vi "Test Array Add.vi"() -> ()   [LabVIEW 2021]
uses:
  Source/Variable/Double Float/Double Float.lvclass
  Source/Variable/Double Float Array/Double Float Array 1D.lvclass
  C:/Users/Tim/Documents/LabVIEW/2021/Data Classes/Source/Element/Vector Parent/Vector Parent.lvclass
  Source/Element/Vector Parent/Vector Parent.lvclass/Vector Parent.ctl
  Source/Element/Vector Parent/Properties/Write Size.vi
  Source/Element/Vector Parent/Properties/Read Index.vi
panel:
  out "Index":i32
  out "Valid Index":bool
  in  "Numeric 2":dbl=1.0
  out "Numeric":dbl
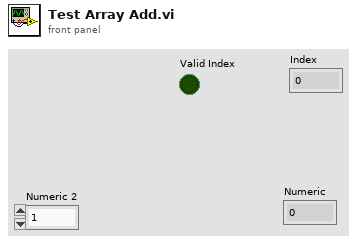
[diagram p1: front panel]
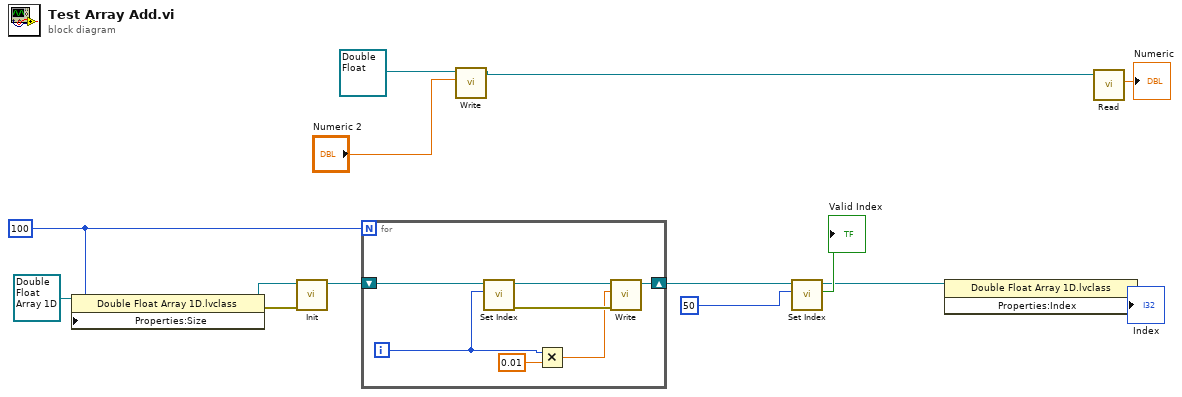
[diagram p0: block diagram]
diagram:
  w5 = 100
  n1 = property class="Double Float Array 1D.lvclass"(reference=refnum<class "Double Float Array 1D.lvclass"> refnum ("Variable.lvlib:Numeric Array.lvclass"), "Properties:Size"=w5) -> (reference out=w6:refnum<class "Double Float Array 1D.lvclass">, error out=w8:errorcluster)  [unwired: 1 in]
  n2 = call-dynamic "Init.vi"("error in (no error)"=w8, "Data in"=w6) -> ("Data out"=w11:refnum<class "Double Float Array 1D.lvclass">)  [unwired: 8 in, 1 out]
  n3 = for {
    N: w5 -> [_]
    shift-right: [w21] -> w10
    shift-left: w11 -> [w20]
    i -> [w17]
    n4 = call-dynamic "Set Index.vi"("Index"=w17, "Array in"=w20) -> ("error out"=w18:errorcluster, "Array out"=w19:refnum<class "Double Float Array 1D.lvclass">)  [unwired: 7 in, 1 out]
    n5 = Multiply(x=w17, y=0.01) -> (x*y=w15:dbl)
    n6 = call-dynamic "Write.vi"("error in (no error)"=w18, "Numeric"=w15, "Numeric Array in"=w19) -> ("Numeric Array out"=w21:refnum<class "Double Float Array 1D.lvclass">)  [unwired: 7 in, 1 out]
  }
  n7 = call-dynamic "Write.vi"("Numeric"="Numeric 2", "Numeric Variable in"=refnum<class "Double Float.lvclass"> refnum ("Variable.lvlib:Numeric.lvclass")) -> ("Numeric Variable out"=w1:refnum<class "Double Float.lvclass">)  [unwired: 8 in, 1 out]
  n8 = call-dynamic "Set Index.vi"("Index"=50, "Array in"=w10) -> ("In Range?"=→"Valid Index":bool, "Array out"=w2:refnum<class "Double Float Array 1D.lvclass">)  [unwired: 7 in, 1 out]
  n9 = property class="Double Float Array 1D.lvclass"(reference=w2) -> ("Properties:Index"=→"Index":i32)  [unwired: 1 in, 2 out]
  n10 = call-dynamic "Read.vi"("Numeric Variable in"=w1) -> ("Numeric"=→"Numeric":dbl)  [unwired: 8 in, 2 out]
